vi "[Example] Send Test Results to Slack Channel.vi"() -> ()   [LabVIEW 2018]
uses:
  Slack API/Slack API.lvlib
panel:
  in  "DUT Part Number":string
  in  "API token":string
  in  "Channel":string
  out "Pass":bool
  out "DUT Measurement":dbl[][](graph)
  # "Slack Workspace"
  # "Getting Started\n\nSlack\n1. Create or find your Slack workspace (https://slack.com/get-started)\n2. Create a bot and save the bot's API token somewhere (https://api.slack.com/bot-users).  Use this API token in this VI.\n3. Create a new channel in your Slack workspace if necessary.  In this VI, specify the Slack channel you want this VI to send a message or image.\n\nPython\n1. Install slackclient v2.0.0 using the \"pip install slackclient=2.0.0\" command."
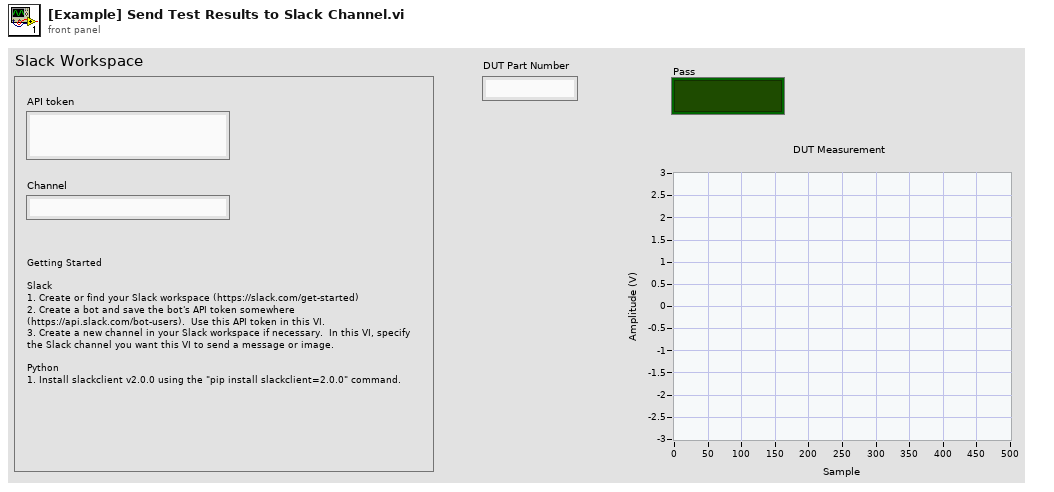
[diagram p1: front panel]
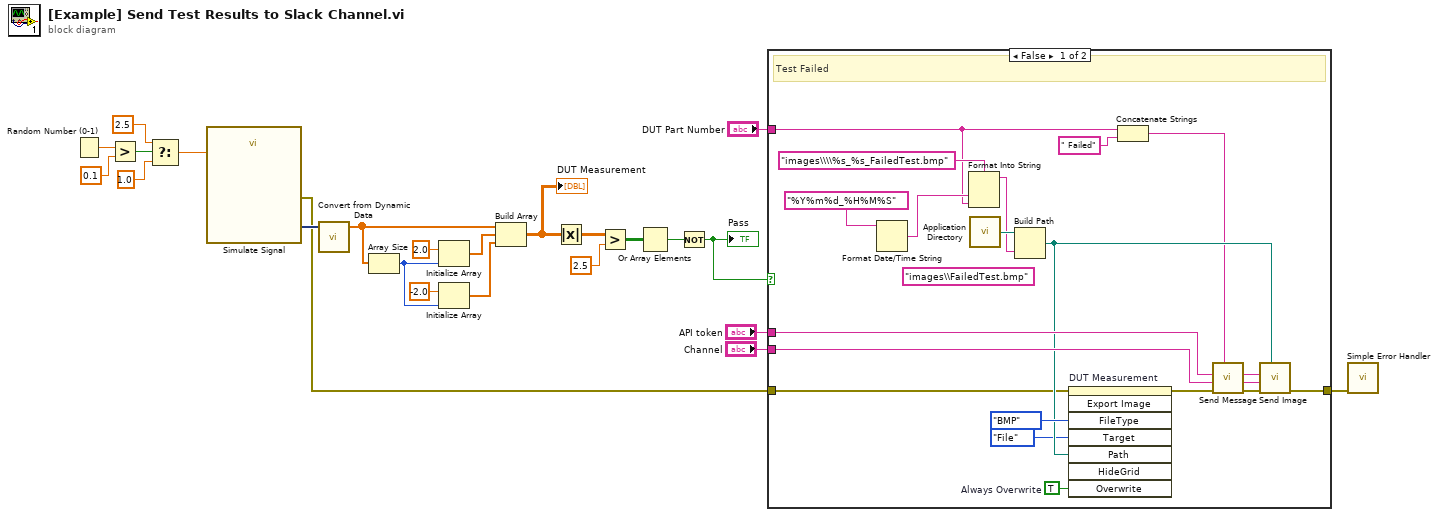
[diagram p0: block diagram]
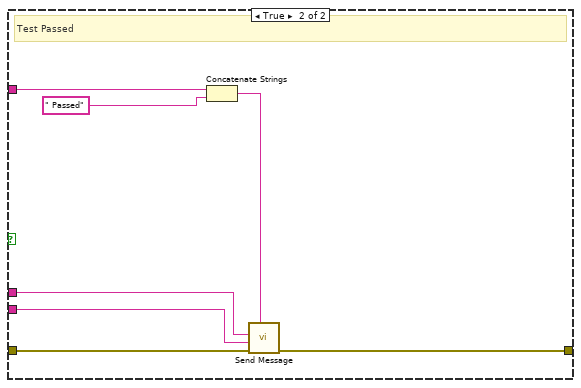
[diagram p2: hidden frame]
diagram:
  n1 = Random Number (0-1)() -> (number: 0 to 1=w17:dbl)
  n2 = Greater?(x=w17, y=0.1) -> (0:w14:bool)
  n3 = Select(t=2.5 ("Amplitude"), s=w14, f=1.0) -> (s? t:f=w13:dbl)
  n4 = call "Simulate Signal"("Amplitude"=w13) -> ("Sine with Uniform Noise"=w24:dynamicdata, "error out"=w3:errorcluster)  [unwired: 13 in]
  n5 = call "Convert from Dynamic Data"("Dynamic Data Type"=w24) -> ("Array"=w23:dbl[])  [unwired: 3 in]
  n6 = Array Size(array=w23) -> (size(s)=w18:i32)
  n7 = Initialize Array(2.0 ("element"), w18) -> (w20:dbl[])
  n8 = Initialize Array(-2.0 ("element"), w18) -> (w19:dbl[])
  n9 = Build Array(w23, w20, w19) -> (w11:dbl[][])
  "DUT Measurement" <- w11
  n10 = Absolute Value(x=w11) -> (abs(x)=w10:dbl[][])
  n11 = Greater?(x=w10, y=2.5 ("element")) -> (0:w8:bool[][])
  n12 = Or Array Elements(Boolean array=w8) -> (logical OR=w7:bool)
  n13 = Not(x=w7) -> (.not. x?=w6:bool)
  "Pass" <- w6
  n14 = case shown="False" w6 {
    tunnel: "API token" -> [w42 w49]
    tunnel: "Channel" -> [w41 w48]
    tunnel: w3 -> [w34 w51]
    tunnel: [w35 w50] -> w2
    tunnel: "DUT Part Number" -> [w25 w46]
    frame False {
      w30 = TRUE  # Always Overwrite
      (unwired) "images\\FailedTest.bmp" ("name or relative path")
      # "Test Failed"
      n15 = Format Date/Time String(time format string (%c)="%Y%m%d_%H%M%S" ("format string")) -> (date/time string=w26:string)  [unwired: 2 in]
      n16 = Format Into String(format string="images\\\\%s_%s_FailedTest.bmp", w26, w25) -> (resulting string=w27:string)  [unwired: 2 in, 1 out]
      n17 = call <vilib>:"Application Directory.vi"() -> ("Application Directory"=w44:path)
      n18 = Build Path(base path=w44, name or relative path=w27) -> (appended path=w37:path)
      n19 = invoke on="DUT Measurement" class="WFGraph (strict)" method="Export Image"(error in=w34, "FileType"=enum32{"BMP", "EPS", "EMF", "PICT"}."BMP" ("File Type"), "Target"=enum32{"File", "Clipboard"}."File", "Path"=w37, "Overwrite"=w30) -> (error out=w33:errorcluster)  [unwired: 3 in, 7 out]
      n20 = Concatenate Strings(w25, " Failed" ("string")) -> (w31:string)
      n21 = call "Send Message.vi"("message"=w31, "error in (no error)"=w33, "slack channel"=w41, "slack API token"=w42) -> ("error out"=w38:errorcluster, "slack channel dup"=w39:string, "slack API token dup"=w40:string)  [unwired: 5 in]
      n22 = call "Send Image.vi"("image filepath"=w37, "error in (no error)"=w38, "slack channel"=w39, "slack API token"=w40) -> ("error out"=w35:errorcluster)  [unwired: 5 in, 2 out]
    }
    frame True {
      # "Test Passed"
      n23 = Concatenate Strings(w46, " Passed" ("string")) -> (w45:string)
      n24 = call "Send Message.vi"("message"=w45, "error in (no error)"=w51, "slack channel"=w48, "slack API token"=w49) -> ("error out"=w50:errorcluster)  [unwired: 5 in, 2 out]
    }
  }
  n25 = call <vilib>:"Simple Error Handler.vi"("error in (no error)"=w2) -> ()  [unwired: 4 in, 5 out]
